vi "Wait on Last Clone Instance Notification.vi"   [LabVIEW 2022 SP3, in "My Cloneable Module.lvlib" / "Clone Registration.lvlib"]
doc: "Wait until the last instance of a cloneable module is stopped.\n_____\nBased on DQMH Project Template 7.0.1.1316."
uses:
  Clone Registration.lvlib
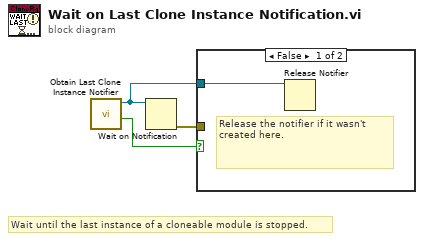
[diagram p0: block diagram]
diagram:
  # "Wait until the last instance of a cloneable module is stopped."
  n1 = call "Obtain Last Clone Instance Notifier.vi"() -> ("created new?"=w3:bool, "Last Instance Notifier"=w2:refnum<notifier>)  [unwired: 10 in]
  n2 = Wait on Notification(notifier=w2) -> (error out=w1:errorcluster)  [unwired: 3 in, 3 out]
  n3 = case shown="False" w3 {
    tunnel: w2 -> [w4 _]
    tunnel: w1 -> [_ _]
    frame False {
      # "Release the notifier if it wasn't created here."
      n4 = Release Notifier(notifier=w4) -> ()  [unwired: 2 in, 3 out]
    }
    frame True {
    }
  }
